vi "Test Load Snapshot - all.vi"() -> (0 "error out":errorcluster)   [LabVIEW 2020]
doc: "Test loading snapshot with breakpoints and probes."
uses:
  src/Path Getter Mock/Path Getter Mock.lvclass
  C:/Users/juanj/Documents/hasbun_wood_engineering/github/Debug-Snapshots-for-LabVIEW/src/IPath Getter/IPath Getter.lvclass
  src/Type Definitions/Snapshot Handling Options--cluster.ctl
  src/Type Definitions/Class Name--enum.ctl
  src/Type Definitions/Debug Snapshot--cluster.ctl
  src/Type Definitions/Breakpoint--cluster.ctl
  <vilib>/Utility/miscctls.llb/LVBreakpointStatusEnum.ctl
  <vilib>/addons/_JKI Toolkits/Caraya/classes/Test/Test.lvclass
  src/Public API.lvlib
  <vilib>/addons/_JKI Toolkits/Caraya/classes/Assert/Assert.lvclass
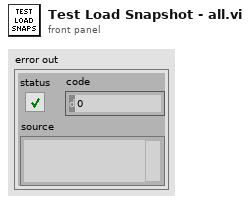
[diagram p1: front panel]
types:
  T1 = typedef "Debug Snapshot--cluster.ctl" = cluster{"VI Name":string, "Breakpoints":T2[], "Probes":i32[]}
  T2 = typedef "Breakpoint--cluster.ctl" = cluster{"UID":i32, "BP Status":T3, "Class Name":T4}
  T3 = typedef "LVBreakpointStatusEnum.ctl" = enum8{"Cleared Break", "Enabled Break", "Disabled Break"}
  T4 = typedef "Class Name--enum.ctl" = enum16{"Node", "Wire"}
  T5 = typedef "Snapshot Handling Options--cluster.ctl" = cluster{"Breakpoints":bool, "Probes":bool}
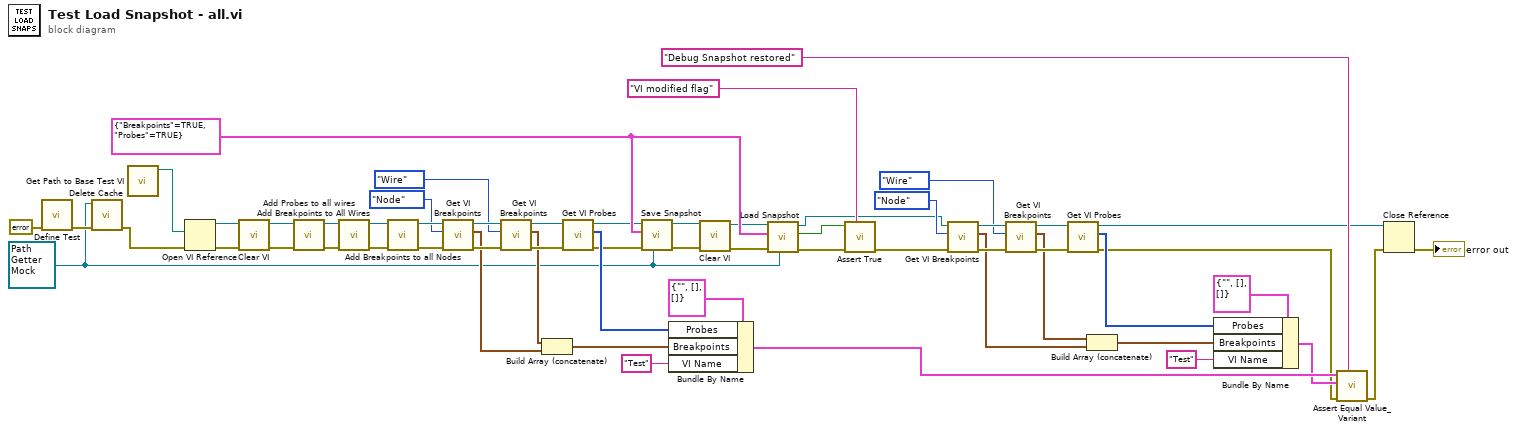
[diagram p0: block diagram]
diagram:
  w46 = T5 {"Breakpoints"=TRUE, "Probes"=TRUE} ("Debug Elements Options")
  w6 = refnum<class "Path Getter Mock.lvclass"> refnum ("Path Getter Mock.lvclass")
  n1 = call <vilib>:"Define Test.vi"("error in (no error)"=errorcluster {"status"=FALSE, "code"=0, "source"=""}) -> ("error out"=w56:errorcluster)  [unwired: 9 in, 1 out]
  n2 = call "Delete Cache.vi"("error in"=w56, "IPath Getter.lvclass"=w6) -> ("error out"=w53:errorcluster)  [unwired: 9 in]
  n3 = call "Get Path to Base Test VI.vi"() -> ("Path"=w54:path)  [unwired: 11 in]
  n4 = Open VI Reference(vi path=w54, error in (no error)=w53) -> (vi reference=w4:refnum<vi>, error out=w55:errorcluster)  [unwired: 4 in]
  n5 = call "Clear VI.vi"("error in"=w55, "VI Refnum In"=w4) -> ("error out"=w5:errorcluster, "VI Refnum Out"=w3:refnum<vi>)  [unwired: 8 in]
  n6 = call "Add Probes to all wires.vi"("error in"=w5, "VI Refnum In"=w3) -> ("error out"=w51:errorcluster, "VI Refnum Out"=w52:refnum<vi>)  [unwired: 8 in]
  n7 = call "Add Breakpoints to All Wires.vi"("error in"=w51, "VI Refnum In"=w52) -> ("error out"=w49:errorcluster, "VI Refnum Out"=w50:refnum<vi>)  [unwired: 8 in]
  n8 = call "Add Breakpoints to all Nodes.vi"("error in"=w49, "VI Refnum In"=w50) -> ("error out"=w44:errorcluster, "VI Refnum Out"=w45:refnum<vi>)  [unwired: 8 in]
  n9 = call "Get VI Breakpoints.vi"("error in"=w44, "Class Name"=Class_Name--enum."Node", "VI Reference in"=w45) -> ("error out"=w42:errorcluster, "Breakpoints"=w37:T2[], "VI Reference out"=w43:refnum<vi>)  [unwired: 6 in]
  n10 = call "Get VI Breakpoints.vi"("error in"=w42, "Class Name"=Class_Name--enum."Wire", "VI Reference in"=w43) -> ("error out"=w40:errorcluster, "Breakpoints"=w36:T2[], "VI Reference out"=w41:refnum<vi>)  [unwired: 6 in]
  n11 = Build Array (concatenate)(w36, w37) -> (w32:T2[])
  n12 = call "Get VI Probes.vi"("error in"=w40, "VI Reference in"=w41) -> ("error out"=w30:errorcluster, "Probes"=w33:i32[], "VI Reference out"=w31:refnum<vi>)  [unwired: 7 in]
  n13 = call "Save Snapshot.vi"("IPath Getter in"=w6, "error in"=w30, "Debug Elements Options"=w46, "VI Reference in"=w31) -> ("error out"=w48:errorcluster, "VI Reference out"=w2:refnum<vi>)  [unwired: 6 in]
  n14 = Bundle By Name(cluster=T1 {"VI Name"="", "Breakpoints"=[], "Probes"=[]} ("Debug Snapshot"), "Probes"=w33, "Breakpoints"=w32, "VI Name"="Test") -> (w12:T1)
  n15 = call "Clear VI.vi"("error in"=w48, "VI Refnum In"=w2) -> ("error out"=w47:errorcluster, "VI Refnum Out"=w1:refnum<vi>)  [unwired: 8 in]
  n16 = call "Load Snapshot.vi"("IPath Getter in"=w6, "error in"=w47, "Debug Elements Options"=w46, "VI Reference in"=w1) -> ("error out"=w22:errorcluster, "VI Modified"=w23:bool, "VI Reference out"=w20:refnum<vi>)  [unwired: 5 in]
  n17 = call <vilib>:"Assert True.vi"("Label"="VI modified flag", "error in (no error)"=w22, "True?"=w23) -> ("error out"=w19:errorcluster)  [unwired: 7 in, 1 out]
  n18 = call "Get VI Breakpoints.vi"("error in"=w19, "Class Name"=Class_Name--enum."Node", "VI Reference in"=w20) -> ("error out"=w28:errorcluster, "Breakpoints"=w13:T2[], "VI Reference out"=w29:refnum<vi>)  [unwired: 6 in]
  n19 = call "Get VI Breakpoints.vi"("error in"=w28, "Class Name"=Class_Name--enum."Wire", "VI Reference in"=w29) -> ("error out"=w26:errorcluster, "Breakpoints"=w14:T2[], "VI Reference out"=w27:refnum<vi>)  [unwired: 6 in]
  n20 = call "Get VI Probes.vi"("error in"=w26, "VI Reference in"=w27) -> ("error out"=w9:errorcluster, "Probes"=w15:i32[], "VI Reference out"=w7:refnum<vi>)  [unwired: 7 in]
  n21 = Build Array (concatenate)(w14, w13) -> (w16:T2[])
  n22 = Bundle By Name(cluster=T1 {"VI Name"="", "Breakpoints"=[], "Probes"=[]} ("Debug Snapshot"), "Probes"=w15, "Breakpoints"=w16, "VI Name"="Test") -> (w11:T1)
  n23 = call <vilib>:"Assert Equal Value_Variant.vi"("Label"="Debug Snapshot restored", "error in (no error)"=w9, "Actual"=w11, "Expected"=w12) -> ("error out"=w8:errorcluster)  [unwired: 6 in, 1 out]
  n24 = Close Reference(reference=w7, error in (no error)=w8) -> (error out=→"error out":errorcluster)
